vi "Stop.vi"(6 "Teller":refnum<class "Teller.lvclass">, 8 "Error in":errorcluster, 11 "Base Actor in":refnum<class "Base Actor.lvclass">) -> (0 "Error out":errorcluster, 3 "Base Actor out":refnum<class "Base Actor.lvclass">)   [LabVIEW 2020, in "jettl.lvlib" / "Base jettl Actor.lvlib" / "Base Actor.lvlib" / "Base Actor.lvclass"]
uses:
  Base Actor.lvclass
  C:/git/jettl/src/jettl/jettl/Actor/Actor.lvclass
  Teller/Teller.lvclass
  Base Actor.lvclass/Base Actor.ctl
  C:/git/jettl/src/jettl/jettl/Base jettl Actor/Base Actor/Base Actor/Base Actor.lvclass
  C:/git/jettl/src/jettl/jettl/Stop jettl Msg/Stop jettl Msg/Stop jettl Msg.lvclass
  C:/git/jettl/src/jettl/jettl/Stopped jettl Msg/Stopped jettl Msg/Stopped jettl Msg.lvclass
  C:/git/jettl/src/jettl/jettl/Stopping jettl Msg/Stopping jettl Msg/Stopping jettl Msg.lvclass
  Lifetime.ctl
  jettl.lvlib
  Stopping jettl Msg/Stopping/Stopping.lvlib
  Stopping jettl Msg/Stopping/Tell Child.vi
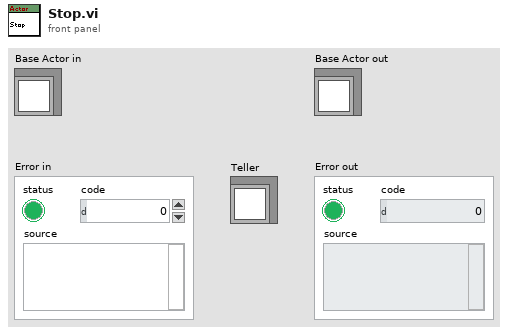
[diagram p1: front panel]
types:
  T1 = typedef "jettl.lvlib/Child UIDs.ctl" = set{string}
  T2 = typedef "jettl.lvlib/Lifetime.ctl" = enum16{"Init", "Spawn", "Pre-Setup", "Setup", "Post-Setup", "Start", "Teardown", "Stopping With Children", "Stopping", "Stopped", "Terminate"}
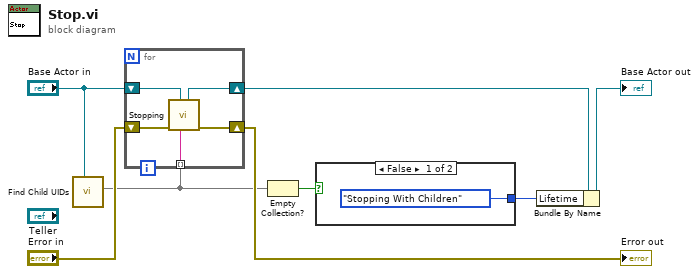
[diagram p0: block diagram]
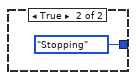
[diagram p2: hidden frame]
diagram:
  n1 = call "Find Child UIDs.vi"("Actor in"="Base Actor in") -> ("Child UIDs"=w3:T1)  [unwired: 10 in]
  n2 = for {
    tunnel: w3 -> [w13] mode=indexing
    shift-right: [w11] -> w7
    shift-left: "Error in" -> [w12]
    shift-right: [w9] -> w1
    shift-left: "Base Actor in" -> [w10]
    n3 = call-poly "Stopping.vi"("UID"=w13, "Actor in"=w10, "Error in"=w12) -> ("Error out"=w11:errorcluster, "Actor out"=w9:refnum<class "Base Actor.lvclass">)  [unwired: 7 in]
  }
  "Error out" <- w7
  n4 = Empty Collection?(1:w3) -> (0:w5:bool)
  n5 = case shown="False" w5 {
    tunnel: [Lifetime."Stopping With Children" ("Lifetime") Lifetime."Stopping" ("Lifetime")] -> w4
    frame False {
    }
    frame True {
    }
  }
  n6 = Bundle By Name(cluster=w1, "Lifetime"=w4) -> (→"Base Actor out":refnum<class "Base Actor.lvclass">)
